vi "IMS Stepper Command.vi"(4 "Timeout Limit":sgl=0.1 format="%.2f", 5 "Motor Number":u32=1 min=1 max=255 step=1, 6 "error in (no error)":errorcluster, 7 "Mode":bool, 8 "Command":string, 9 "Instrument Address":refnum<visa-resource-name>) -> (0 "error out":errorcluster, 1 "Response":string, 2 "Timeout":bool, 3 "Instrument Address Out":refnum<visa-resource-name>)   [LabVIEW 2024]
uses:
  Serial Support VISA.llb/Serial Actions.ctl
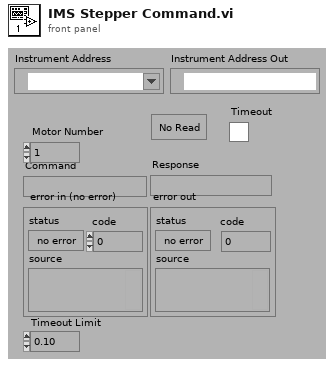
[diagram p1: front panel]
types:
  T1 = typedef "Serial Actions.ctl" = enum16{"Init", "Break", "Clear Buffer", "Write", "Read", "N Bytes", "Lock", "Unlock", "Close"}
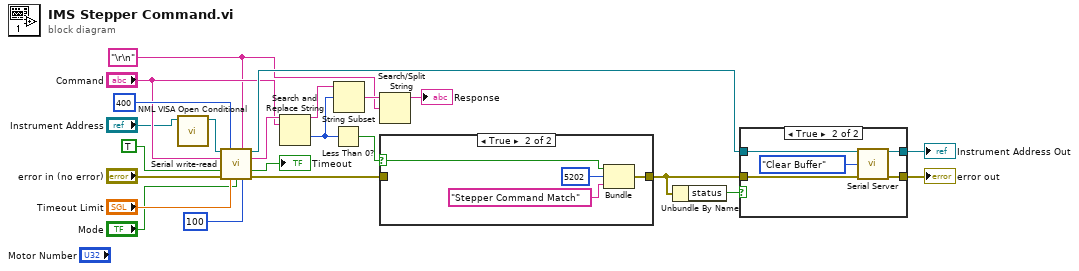
[diagram p0: block diagram]
diagram:
  w4 = "\r\n" ("EOT Chars (cr/lf)")
  n1 = call "NML VISA Open Conditional.vi"("VISA resource name"="Instrument Address") -> ("dup VISA Session"=w1:refnum<visa-resource-name>)  [unwired: 8 in, 2 out]
  n2 = call "Serial write-read.vi"("VISA Resource Name"=w1, "Max Char to Read"=u32 400, "EOT Chars (cr/lf)"=w4, "String To Send"="Command", "Clear Buffer?"=TRUE, "error in (no error)"="error in (no error)", "Timeout Limit"="Timeout Limit", "Read Echo?"="Mode", "milliseconds to wait"=u32 100) -> ("dup VISA Resource Name"=w18:refnum<visa-resource-name>, "Serial Read"=w11:string, "Timeout"=→"Timeout":bool, "error out"=w21:errorcluster)  [unwired: 1 in, 2 out]
  n3 = Search and Replace String(input string=w11, search string="Command") -> (result string=w7:string, offset past replacement=w6:i32)  [unwired: 6 in, 2 out]
  n4 = Less Than 0?(x=w6) -> (x < 0?=w9:bool)
  n5 = String Subset(string=w7, offset (0)=w6) -> (substring=w8:string)  [unwired: 1 in]
  n6 = Search/Split String(string=w8, search string/char (-)=w4) -> (substring before match=→"Response":string)  [unwired: 1 in, 2 out]
  n7 = case shown="True" w9 {
    selector: w9 -> [_ w27]
    tunnel: [w24 w28] -> w13
    tunnel: w21 -> [w24 _]
    frame False {
    }
    frame True {
      n8 = Bundle(w27, 5202, "Stepper Command Match") -> (w28:errorcluster)  [unwired: 1 in]
    }
  }
  n9 = Unbundle By Name(w13) -> ("status"=w22:bool)
  n10 = case shown="True" w22 {
    tunnel: w18 -> [w29 w34]
    tunnel: [w30 w33] -> w14
    tunnel: w13 -> [w30 w32]
    tunnel: [w29 w31] -> w3
    frame False {
    }
    frame True {
      n11 = call "Serial Server.vi"("VISA Resource Name"=w34, "Action"=Serial_Actions."Clear Buffer", "error in (no error)"=w32) -> ("dup VISA Resource Name"=w31:refnum<visa-resource-name>, "error out"=w33:errorcluster)  [unwired: 8 in, 3 out]
    }
  }
  "error out" <- w14
  "Instrument Address Out" <- w3
